vi "number_to_boolean.vi"(1 "A in":i32) -> (0 "A out":bool[](array[boolean]))   [LabVIEW 2020]
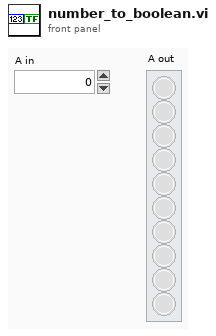
[diagram p1: front panel]
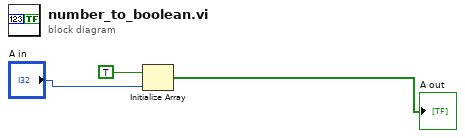
[diagram p0: block diagram]
diagram:
  n1 = Initialize Array "Initialize Array"(TRUE, "A in") -> (→"A out":bool[])
